vi "Compute Friction.vi"(8 "error in (no error)":errorcluster, 10 "qd":dbl, 11 "Link in":refnum<class "Link.lvclass">) -> (0 "error out":errorcluster, 2 "Friction":dbl, 3 "Link out":refnum<class "Link.lvclass">)   [LabVIEW 2013, in "Link.lvclass"]
uses:
  Link.lvclass
  Link.lvclass/Link.ctl
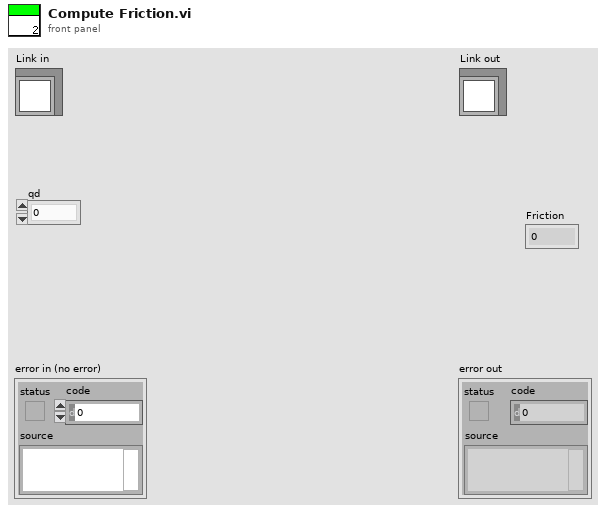
[diagram p1: front panel]
types:
  T1 = cluster{"Positive Movement":dbl, "Negative Movement":dbl}
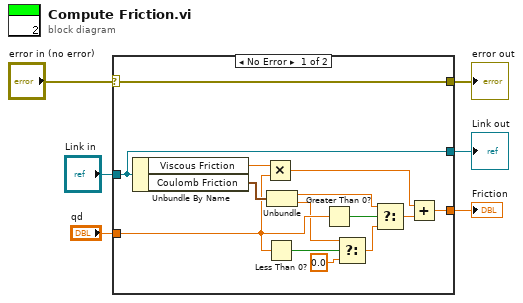
[diagram p0: block diagram]
diagram:
  n1 = case shown="No Error" "error in (no error)" {
    selector: "error in (no error)" -> [w7 w21]
    tunnel: "Link in" -> [w8 w22]
    tunnel: "qd" -> [w18 _]
    tunnel: [w10 _] -> w3
    tunnel: [w8 w22] -> w4
    tunnel: [w7 w21] -> w5
    frame No Error {
      n2 = Unbundle By Name(w8) -> ("Viscous Friction"=w20:dbl, "Coulomb Friction"=w19:T1)
      n3 = Multiply(x=w20, y=w18) -> (x*y=w11:dbl)
      n4 = Less Than 0?(x=w18) -> (x < 0?=w16:bool)
      n5 = Unbundle(w19) -> ("Positive Movement"=w15:dbl, "Negative Movement"=w13:dbl)
      n6 = Greater Than 0?(x=w18) -> (x > 0?=w17:bool)
      n7 = Select(t=w13, s=w16, f=0.0) -> (s? t:f=w14:dbl)
      n8 = Select(t=w15, s=w17, f=w14) -> (s? t:f=w12:dbl)
      n9 = Add(x=w11, y=w12) -> (x+y=w10:dbl)
    }
    frame Error {
    }
  }
  "error out" <- w5
  "Link out" <- w4
  "Friction" <- w3
